vi "Sample Wire Data.vi"() -> ()   [LabVIEW 2017]
uses:
  <vilib>/Utility/file.llb/Write Delimited Spreadsheet (DBL).vi
panel:
  out "Waveform Graph":dynamicdata(graph)
  in  "Overwrite File?":bool=TRUE
  in  "file path (dialog if empty)":path
  in  "Controls":T1={"Sample Rate (Hz)"=5000.0, "Number of Samples"=50000.0}
  out "Error Out":errorcluster
  in  "Error In":errorcluster
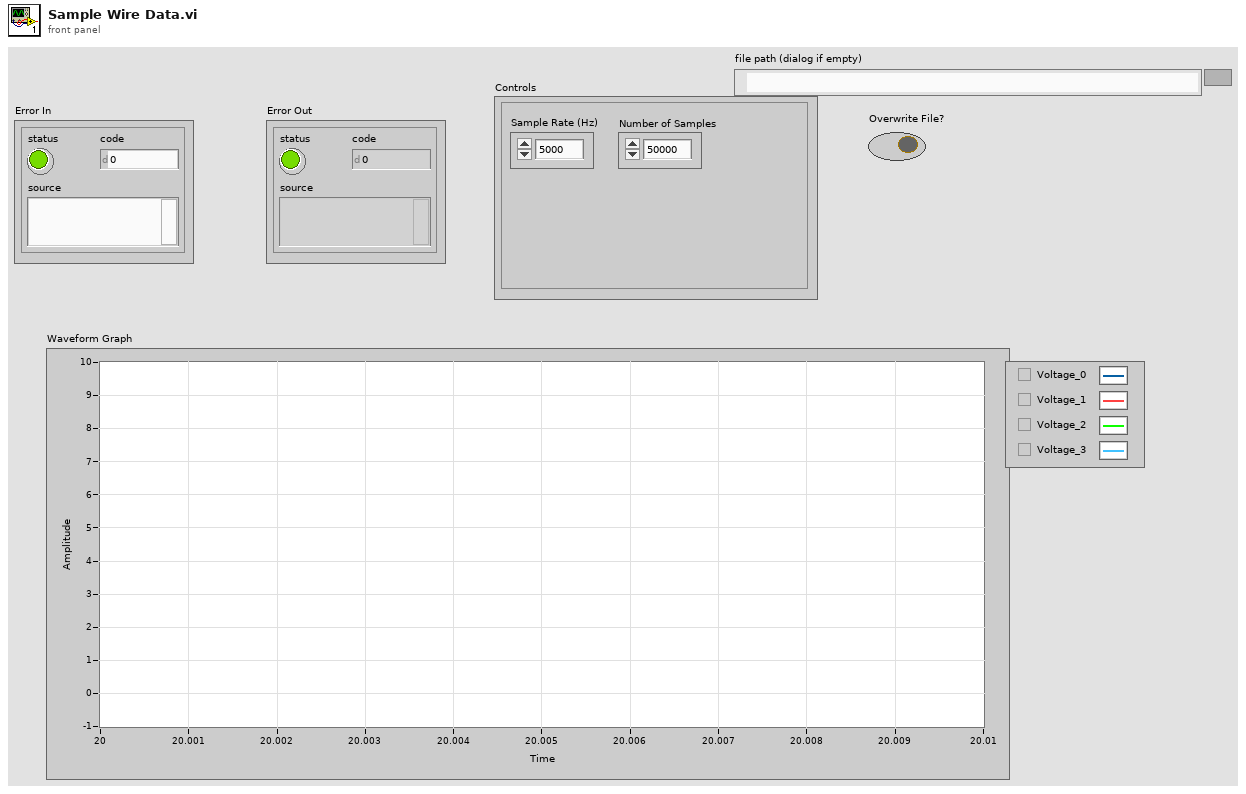
[diagram p1: front panel]
types:
  T1 = cluster{"Sample Rate (Hz)":dbl, "Number of Samples":dbl}
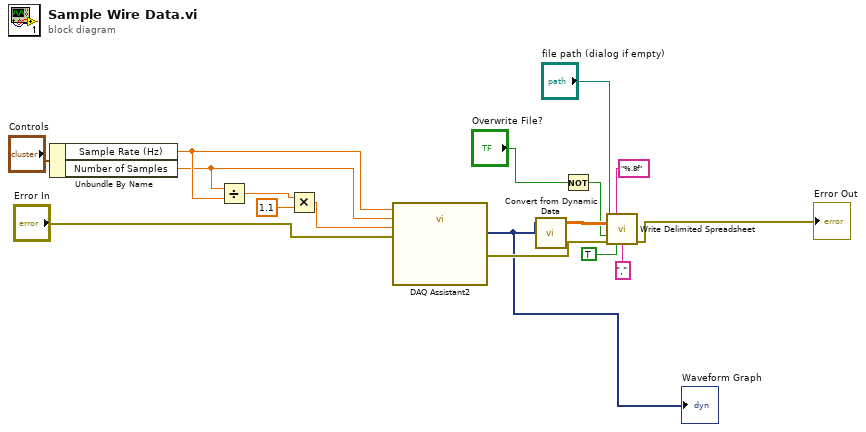
[diagram p0: block diagram]
diagram:
  n1 = Unbundle By Name("Controls") -> ("Sample Rate (Hz)"=w5:dbl, "Number of Samples"=w4:dbl)
  n2 = Divide(x=w4, y=w5) -> (x/y=w16:dbl)
  n3 = Multiply(x=w16, y=1.1) -> (x*y=w6:dbl)
  n4 = call "DAQ Assistant2"("rate"=w5, "number of samples"=w4, "timeout (s)"=w6, "error in"="Error In") -> ("data"=w1:dynamicdata, "error out"=w2:errorcluster)  [unwired: 13 in, 1 out]
  "Waveform Graph" <- w1
  n5 = call "Convert from Dynamic Data"("Dynamic Data Type"=w1) -> ("Array"=w14:dbl[][])  [unwired: 3 in]
  n6 = Not(x="Overwrite File?") -> (.not. x?=w9:bool)
  n7 = call-poly <vilib>:"Write Delimited Spreadsheet.vi"("file path (dialog if empty)"="file path (dialog if empty)", "format (%.3f)"="%.8f", "2D data"=w14, "append to file? (new file:F)"=w9, "error in (no error)"=w2, "transpose? (no:F)"=TRUE, "delimiter (\\t)"="," ("delimiter (\\t)")) -> ("error out"=→"Error Out":errorcluster)  [unwired: 7 in, 1 out]
